vi "简单内置对话框演示.vi"() -> ()   [LabVIEW 2013]
panel:
  in  "退出":bool
  in  "启用":bool
  in  "显示对话框":bool
  in  "三按钮对话框":bool
  in  "双按钮对话框":bool
  in  "单按钮对话框":bool
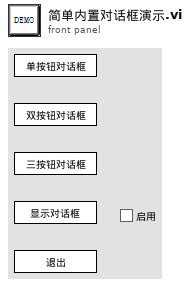
[diagram p1: front panel]
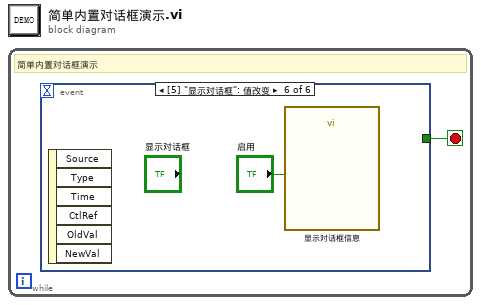
[diagram p0: block diagram]
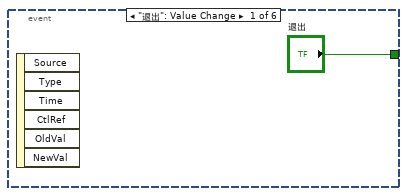
[diagram p2: hidden frame]
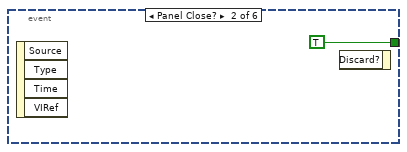
[diagram p3: hidden frame]
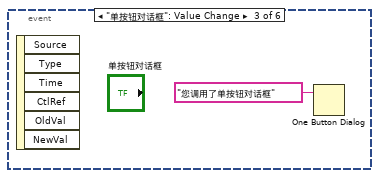
[diagram p4: hidden frame]
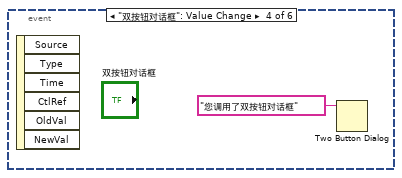
[diagram p5: hidden frame]
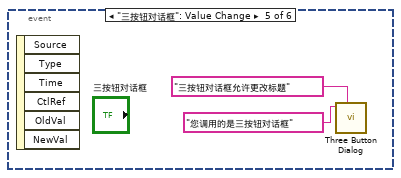
[diagram p6: hidden frame]
diagram:
  n1 = while {
    stop <- w1 stop-if-true
    # "简单内置对话框演示"
    n2 = event shown="[5] \"显示对话框\": 值改变" {
      selector: _ -> [_ _ _ _ _ _]
      dyn-events: _ -> [_ _ _ _ _ _]
      timeout: _ -> [_ _ _ _ _ _]
      tunnel: ["退出" TRUE ("退出") _ _ _ _] -> w1
      event "退出": Value Change {
        n3 = event-data() -> ()  [unwired: 1 in, 6 out]
      }
      event Panel Close? {
        n4 = event-data() -> ()  [unwired: 1 in, 4 out]
        n5 = event-data() -> ()  [unwired: 2 in, 1 out]
      }
      event "单按钮对话框": Value Change {
        n6 = event-data() -> ()  [unwired: 1 in, 6 out]
        n7 = One Button Dialog(message="您调用了单按钮对话框" ("消息")) -> ()  [unwired: 1 in, 1 out]
      }
      event "双按钮对话框": Value Change {
        n8 = event-data() -> ()  [unwired: 1 in, 6 out]
        n9 = Two Button Dialog(message="您调用了双按钮对话框" ("消息")) -> ()  [unwired: 2 in, 1 out]
      }
      event "三按钮对话框": Value Change {
        n10 = event-data() -> ()  [unwired: 1 in, 6 out]
        n11 = call <vilib>:"Three Button Dialog.vi"("Window Title (\"\")"="三按钮对话框允许更改标题" ("Window Title (\"\")"), "message"="您调用的是三按钮对话框") -> ()  [unwired: 9 in, 1 out]
      }
      event "显示对话框": Value Change {
        n12 = event-data() -> ()  [unwired: 1 in, 6 out]
        n13 = call "显示对话框信息"("Enable"="启用") -> ()  [unwired: 9 in, 2 out]
      }
    }
  }
